vi "Fetch Multi Eval Meas List ES Flatness Ripple Results.vi"(6 "Ripple (Ripple 1)":T1=1 items=["Ripple 1"=1, "Ripple 2"=2], 8 "error in (no error)":errorcluster, 9 "Result Type (Current)":i32(ring) items=["Current", "Average", "Extreme", "Standard Deviation"], 10 "Instance (1)":T2=1, 11 "VISA resource name":refnum<visa-resource-name>) -> (0 "error out":errorcluster, 1 "Results":dbl[](array[numeric]) format="%^.3e", 2 "Reliability":i32, 3 "VISA resource name out":refnum<visa-resource-name>)   [LabVIEW 2020, in "Rohde&Schwarz CMWXP NR FR1 Measurement.lvlib"]
doc: "Return equalizer spectrum flatness single value results (ripple 1 or ripple 2) for all measured list mode segments.\n\nAttributes:\nRSCMWXPNRFR1M_ATTR_FETCH_MULTI_EVAL_MEAS_LIST_ES_FLATNESS_RIPPLE_CURRENT_RESULTS\nRSCMWXPNRFR1M_ATTR_FETCH_MULTI_EVAL_MEAS_LIST_ES_FLATNESS_RIPPLE_AVERAGE_RESULTS\nRSCMWXPNRFR1M_ATTR_FETCH_MULTI_EVAL_MEAS_LIST_ES_FLATNESS_RIPPLE_EXTREME_RESULTS\nRSCMWXPNRFR1M_ATTR_FETCH_MULTI_EVAL_MEAS_LIST_ES_FLATNESS_RIPPLE_STANDARD_DEVIATION_RESULTS\n\nRemote-control commands:\nFETCh:NRSub:MEAS<i>:MEValuation:LIST:ESFLatness:RIPPle<no>:CURRent?\nFETCh:NRSub:MEAS<i>:MEValuation:LIST:ESFLatness:RIPPle<no>:AVERage?\nFETCh:NRSub:MEAS<i>:MEValuation:LIST:ESFLatness:RIPPle<no>:EXTReme?\nFETCh:NRSub:MEAS<i>:MEValuation:LIST:ESFLatness:RIPPle<no>:SDEViation?"
uses:
  <instrlib>/Rohde&Schwarz CMWXP NR FR1 Measurement/Rohde&Schwarz CMWXP NR FR1 Measurement.lvlib
  <instrlib>/Rohde&Schwarz CMWXP NR FR1 Measurement/Private/_Instance.ctl
  <instrlib>/Rohde&Schwarz CMWXP NR FR1 Measurement/Private/_Ripple.ctl
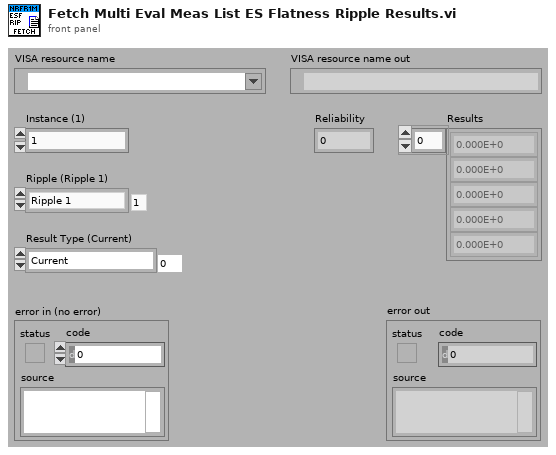
[diagram p1: front panel]
types:
  T1 = typedef "Rohde&Schwarz CMWXP NR FR1 Measurement.lvlib/_Ripple.ctl" = i32
  T2 = typedef "Rohde&Schwarz CMWXP NR FR1 Measurement.lvlib/_Instance.ctl" = i32
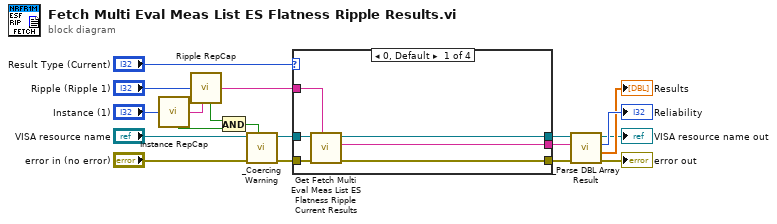
[diagram p0: block diagram]
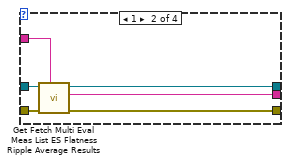
[diagram p2: hidden frame]
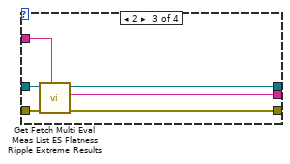
[diagram p3: hidden frame]
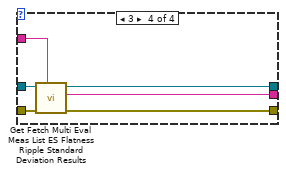
[diagram p4: hidden frame]
diagram:
  n1 = call <instrlib>:"Instance RepCap.vi"("Instance In"="Instance (1)") -> ("In Range?"=w14:bool, "RepCap Identifier Out"=w13:string)  [unwired: 1 in]
  n2 = call <instrlib>:"Ripple RepCap.vi"("Ripple In"="Ripple (Ripple 1)", "RepCap String In (\"\")"=w13) -> ("In Range?"=w12:bool, "RepCap Identifier Out"=w11:string)
  n3 = And(x=w12, y=w14) -> (x .and. y?=w15:bool)
  n4 = call <instrlib>:"_Coercing Warning.vi"("In Range?"=w15, "error in (no error)"="error in (no error)", "VISA resource name"="VISA resource name") -> ("error out"=w9:errorcluster, "VISA resource name out"=w10:refnum<visa-resource-name>)  [unwired: 7 in]
  n5 = case shown="0, Default" "Result Type (Current)" {
    tunnel: w11 -> [w25 w31 w37 w43]
    tunnel: w10 -> [w24 w30 w36 w42]
    tunnel: w9 -> [w23 w29 w35 w41]
    tunnel: [w22 w28 w34 w40] -> w5
    tunnel: [w21 w27 w33 w39] -> w6
    tunnel: [w20 w26 w32 w38] -> w7
    frame 0, Default {
      n6 = call "Get Fetch Multi Eval Meas List ES Flatness Ripple Current Results"("Repeated Capabilities"=w25, "error in (no error)"=w23, "instrument handle"=w24) -> ("error out"=w20:errorcluster, "Fetch Multi Eval Meas List ES Flatness Ripple Current Results"=w21:string, "instrument handle out"=w22:refnum<visa-resource-name>)  [unwired: 6 in]
    }
    frame 1 {
      n7 = call "Get Fetch Multi Eval Meas List ES Flatness Ripple Average Results"("Repeated Capabilities"=w31, "error in (no error)"=w29, "instrument handle"=w30) -> ("error out"=w26:errorcluster, "Fetch Multi Eval Meas List ES Flatness Ripple Average Results"=w27:string, "instrument handle out"=w28:refnum<visa-resource-name>)  [unwired: 6 in]
    }
    frame 2 {
      n8 = call "Get Fetch Multi Eval Meas List ES Flatness Ripple Extreme Results"("Repeated Capabilities"=w37, "error in (no error)"=w35, "instrument handle"=w36) -> ("error out"=w32:errorcluster, "Fetch Multi Eval Meas List ES Flatness Ripple Extreme Results"=w33:string, "instrument handle out"=w34:refnum<visa-resource-name>)  [unwired: 6 in]
    }
    frame 3 {
      n9 = call "Get Fetch Multi Eval Meas List ES Flatness Ripple Standard Deviation Results"("Repeated Capabilities"=w43, "error in (no error)"=w41, "instrument handle"=w42) -> ("error out"=w38:errorcluster, "Fetch Multi Eval Meas List ES Flatness Ripple Standard Deviation Results"=w39:string, "instrument handle out"=w40:refnum<visa-resource-name>)  [unwired: 6 in]
    }
  }
  n10 = call <instrlib>:"_Parse DBL Array Result.vi"("error in (no error)"=w7, "Input String"=w6, "VISA resource name"=w5) -> ("error out"=→"error out":errorcluster, "Results"=→"Results":dbl[], "Reliability"=→"Reliability":i32, "VISA resource name out"=→"VISA resource name out":refnum<visa-resource-name>)  [unwired: 5 in]
